vi "Probability.vi"(1 "MODE":i32(knob) scale=0.0..2.0) -> (0 "flip":bool)   [LabVIEW 2013]
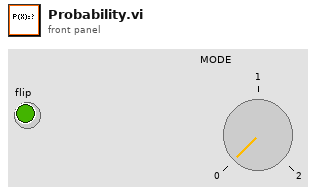
[diagram p1: front panel]
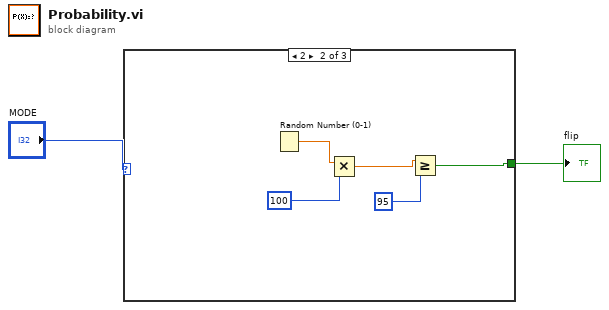
[diagram p0: block diagram]
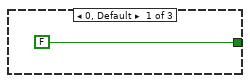
[diagram p2: hidden frame]
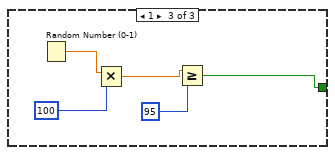
[diagram p3: hidden frame]
diagram:
  n1 = case shown="2" "MODE" {
    tunnel: [FALSE w4 w9] -> w1
    frame 0, Default {
    }
    frame 2 {
      n2 = Random Number (0-1)() -> (number: 0 to 1=w8:dbl)
      n3 = Multiply(x=w8, y=100) -> (x*y=w6:dbl)
      n4 = Greater Or Equal?(x=w6, y=95) -> (x >= y?=w4:bool)
    }
    frame 1 {
      n5 = Random Number (0-1)() -> (number: 0 to 1=w13:dbl)
      n6 = Multiply(x=w13, y=100) -> (x*y=w11:dbl)
      n7 = Greater Or Equal?(x=w11, y=95) -> (x >= y?=w9:bool)
    }
  }
  "flip" <- w1
